vi "Write Spectral Data TDMS (SubVI).vi"(0 "tdms file":refnum<k34>, 1 "Loop Iteration":i32, 2 "Time Stamp":timestamp, 3 "Shutter":bool=TRUE, 4 "Write Spectral Data":bool, 5 "error in (no error)":errorcluster, 6 "Data":dbl[](array[numeric]), 11 "Flush Freq":i32) -> (14 "tdms file 2":refnum<k34>, 19 "error out":errorcluster)   [LabVIEW 2018]
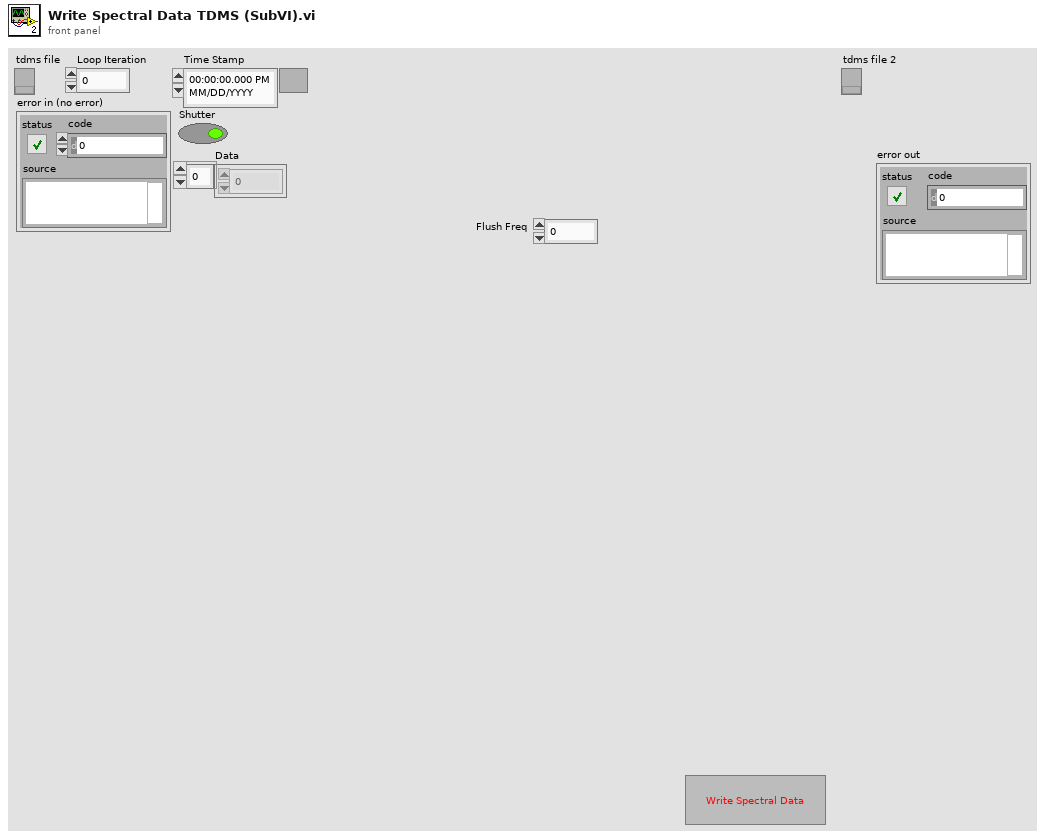
[diagram p1: front panel]
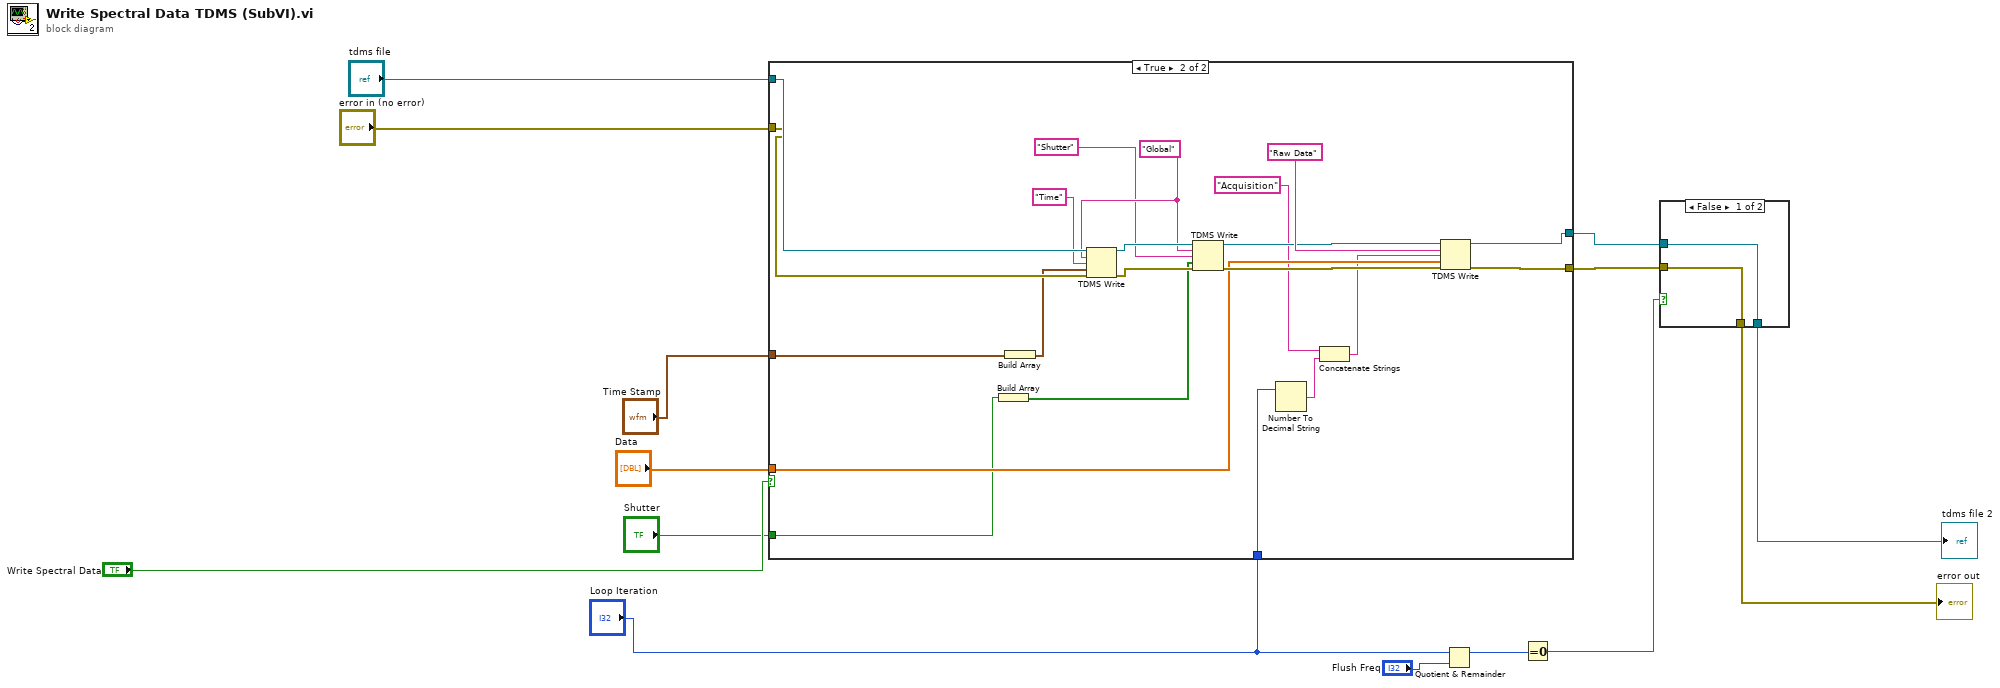
[diagram p0: block diagram]
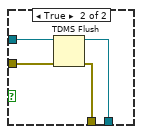
[diagram p2: hidden frame]
diagram:
  n1 = case shown="True" "Write Spectral Data" {
    tunnel: "tdms file" -> [w16 w30]
    tunnel: "error in (no error)" -> [w15 w29]
    tunnel: [w15 w32] -> w10
    tunnel: [w16 w31] -> w9
    tunnel: "Data" -> [_ w27]
    tunnel: "Time Stamp" -> [_ w26]
    tunnel: "Shutter" -> [_ w24]
    tunnel: "Loop Iteration" -> [_ w19]
    frame False {
    }
    frame True {
      w28 = "Global" ("group name in (Untitled)")
      n2 = Build Array(w24) -> (w22:bool[])
      n3 = Build Array(w26) -> (w25:timestamp[])
      n4 = TDMS Write(0:w30, 5:w28, 7:"Time" ("group name in (Untitled)"), 9:w25, 11:w29) -> (4:w36:refnum<k34>, 15:w34:errorcluster)  [unwired: 1 in, 2 out]
      n5 = TDMS Write(0:w36, 5:w28, 7:"Shutter" ("group name in (Untitled)"), 9:w22, 11:w34) -> (4:w35:refnum<k34>, 15:w33:errorcluster)  [unwired: 1 in, 2 out]
      n6 = Number To Decimal String(number=w19) -> (decimal integer string=w18:string)  [unwired: 1 in]
      n7 = Concatenate Strings("Acquisition" ("group name in (Untitled)"), w18) -> (w17:string)
      n8 = TDMS Write(0:w35, 5:"Raw Data" ("group name in (Untitled)"), 7:w17, 9:w27, 11:w33) -> (4:w31:refnum<k34>, 15:w32:errorcluster)  [unwired: 1 in, 2 out]
    }
  }
  n9 = Quotient & Remainder(x="Loop Iteration", y="Flush Freq") -> (x-y*floor(x/y)=w6:i32)  [unwired: 1 out]
  n10 = Equal To 0?(x=w6) -> (x = 0?=w5:bool)
  n11 = case shown="False" w5 {
    tunnel: w10 -> [w38 w43]
    tunnel: w9 -> [w39 w42]
    tunnel: [w38 w41] -> w8
    tunnel: [w39 w40] -> w7
    frame False {
    }
    frame True {
      n12 = TDMS Flush(4:w43, 7:w42) -> (0:w41:errorcluster, 3:w40:refnum<k34>)
    }
  }
  "tdms file 2" <- w7
  "error out" <- w8
